vi "Set Transfer Configurations.vi"(10 "Transfer Configurations":refnum<class "Transfer Configuration.lvclass">[](array[class]), 11 "Transfer Group Configuration in":refnum<class "Transfer Group Configuration.lvclass">) -> (3 "Transfer Group Configuration out":refnum<class "Transfer Group Configuration.lvclass">)   [LabVIEW 2017, in "Data Sharing Framework Core.lvlib" / "Data Sharing Framework Engine.lvlib" / "Transfer Group Configuration.lvclass"]
uses:
  Transfer Group Configuration.lvclass
  Transfer Configuration/Transfer Configuration.lvclass
  Transfer Group Configuration.lvclass/Transfer Group Configuration.ctl
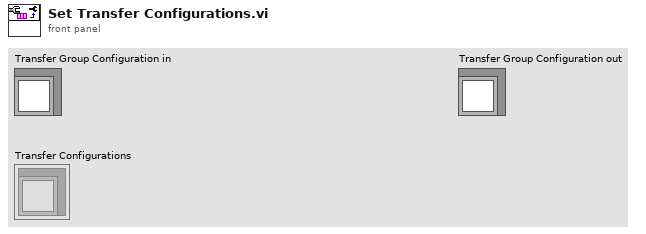
[diagram p1: front panel]
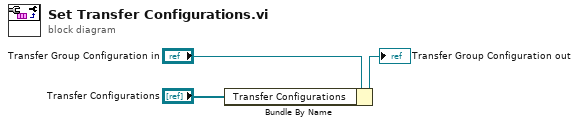
[diagram p0: block diagram]
diagram:
  n1 = Bundle By Name(cluster="Transfer Group Configuration in", "Transfer Configurations"="Transfer Configurations") -> (→"Transfer Group Configuration out":refnum<class "Transfer Group Configuration.lvclass">)
